vi "Text file pattern_.vi"(8 "error in":errorcluster) -> (0 "error out":errorcluster, 2 "путь к файлу":path)   [LabVIEW 2013]
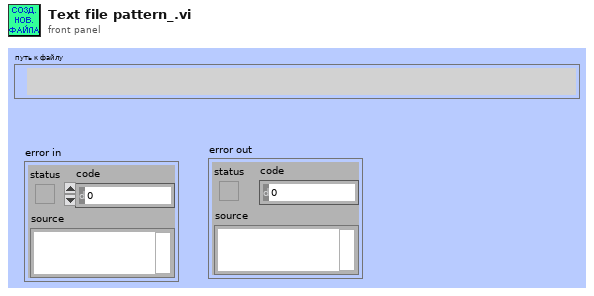
[diagram p1: front panel]
types:
  T1 = enum16{"open", "replace", "create", "open or create", "replace or create", "replace or create with confirmation"}
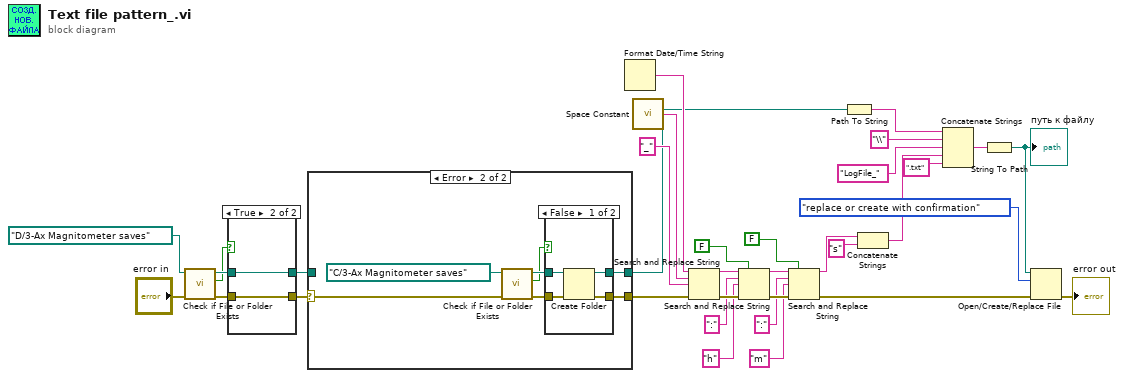
[diagram p0: block diagram]
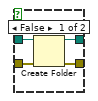
[diagram p4: hidden frame]
diagram:
  n1 = call <vilib>:"Check if File or Folder Exists.vi"("error in (no error)"="error in", "path"=path "D:/3-Ax Magnitometer saves" ("path (use dialog)")) -> ("error out"=w33:errorcluster, "file or folder exists?"=w31:bool, "dup path"=w34:path)  [unwired: 7 out]
  n2 = case shown="True" w31 {
    tunnel: [w38 w40] -> w29
    tunnel: w34 -> [w37 w40]
    tunnel: w33 -> [w36 w39]
    tunnel: [w35 w39] -> w30
    frame False {
      n3 = Create Folder(path (use dialog)=w37, error in=w36) -> (created path=w38:path, error out=w35:errorcluster)  [unwired: 2 out]
    }
    frame True {
    }
  }
  n4 = case shown="Error" w30 {
    selector: w30 -> [w41 w43]
    tunnel: w29 -> [w42 _]
    tunnel: [w42 w46] -> w3
    tunnel: [w41 w45] -> w4
    frame No Error {
    }
    frame Error {
      n5 = call <vilib>:"Check if File or Folder Exists.vi"("error in (no error)"=w43, "path"=path "C:/3-Ax Magnitometer saves" ("path (use dialog)")) -> ("error out"=w48:errorcluster, "file or folder exists?"=w47:bool, "dup path"=w49:path)  [unwired: 7 out]
      n6 = case shown="False" w47 {
        tunnel: [w53 w55] -> w46
        tunnel: w49 -> [w52 w55]
        tunnel: w48 -> [w51 w54]
        tunnel: [w50 w54] -> w45
        frame False {
          n7 = Create Folder(path (use dialog)=w52, error in=w51) -> (created path=w53:path, error out=w50:errorcluster)  [unwired: 2 out]
        }
        frame True {
        }
      }
    }
  }
  n8 = Format Date/Time String() -> (date/time string=w27:string)  [unwired: 3 out]
  n9 = call <vilib>:"Space Constant.vi"() -> ("String"=w7:string)
  n10 = Search and Replace String(input string=w27, search string=w7, replace string="_" ("replace string (\"\")"), error in=w4) -> (result string=w9:string, error out=w19:errorcluster)  [unwired: 6 out]
  n11 = Search and Replace String(replace all?=FALSE ("replace all? (F)"), input string=w9, search string=":", replace string="h" ("replace string (\"\")"), error in=w19) -> (result string=w16:string, error out=w20:errorcluster)  [unwired: 5 out]
  n12 = Search and Replace String(replace all?=FALSE ("replace all? (F)"), input string=w16, search string=":", replace string="m" ("replace string (\"\")"), error in=w20) -> (result string=w22:string, error out=w21:errorcluster)  [unwired: 5 out]
  n13 = Path To String(path=w3) -> (string=w17:string)
  n14 = Concatenate Strings(w22, "s" ("string")) -> (w25:string)
  n15 = Concatenate Strings(w17, "\\" ("string"), "LogFile_" ("string"), w25, ".txt" ("default name")) -> (w6:string)
  n16 = String To Path(string=w6) -> (path=w2:path)
  "путь к файлу" <- w2
  n17 = Open/Create/Replace File(file path (use dialog)=w2, error in=w21, operation (0:open)=T1."replace or create with confirmation") -> (error out=→"error out":errorcluster)  [unwired: 5 out]
